vi "HowForebrainPerception.vi"(1 "How?MidbrainIn":cluster{"T":dbl, "Battey":dbl, "Temp":dbl}) -> (2 "TempWarning":bool, 3 "How?ForebrainOut":cluster{"T":dbl, "Battery":dbl, "Temp":dbl}, 4 "BatteryGauge":dbl)   [LabVIEW 2012]
doc: "This SubVI takes clean How sense data from the Midbrain and layers perception onto it to be passed to the THINK processes in the Forebrain"
panel:
  # "This SubVI adds \nperception onto the\nHow data comming\nfrom the Midbrain"
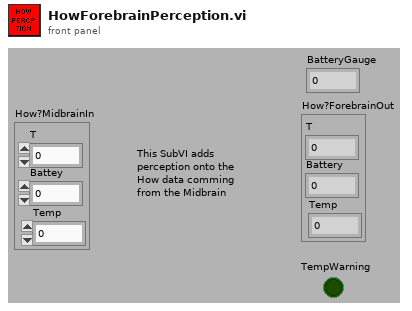
[diagram p1: front panel]
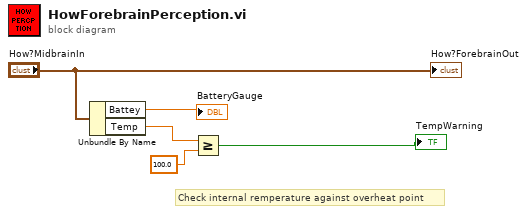
[diagram p0: block diagram]
diagram:
  # "Check internal remperature against overheat point"
  n1 = Unbundle By Name("How?MidbrainIn") -> ("Battey"=→"BatteryGauge":dbl, "Temp"=w3:dbl)
  n2 = Greater Or Equal?(x=w3, y=100.0) -> (x >= y?=→"TempWarning":bool)
  "How?ForebrainOut" <- "How?MidbrainIn"
